vi "Refresh.vi"(0 "reference in":refnum<class "LcPictureBox.lvclass">, 5 "Error In":errorcluster) -> (14 "reference out":refnum<class "LcPictureBox.lvclass">, 19 "Error Out":errorcluster)   [LabVIEW 2020, in "LcPictureBox.lvclass"]
uses:
  LcPictureBox.lvclass
  System.Windows.Forms
  System.Drawing
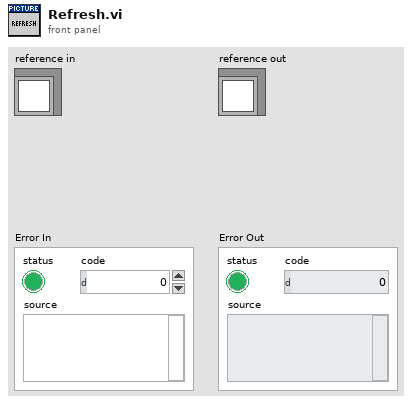
[diagram p1: front panel]
types:
  T1 = typedef "LcPictureBox.lvclass/ObjectAttributes.ctl" = cluster{"PictureBox":refnum<k24>, "ImageSize":cluster{"Width":i32, "Height":i32}, "PenMemory":map{cluster{"Alpha(100%)":dbl, "Color(Black)":u32, "Pen(Width=1, Solid)":T2}, refnum<k24>}, "GraphicsRef":refnum<k24>, "BrushMemory":map{cluster{"Alpha(100%)":dbl, "Color(Black)":u32}, refnum<k24>}, "Images":refnum<k24>[], "ImageIndex":i32, "BgColor(None)":u32, "LoadedImages":map{string, cluster{"ImageOut":refnum<k24>, "ImageSize":cluster{"Width":i32, "Height":i32}}}, "ColorsMemory":map{cluster{"Alpha(100%)":dbl, "Color(Black)":u32}, refnum<k24>}, "CacheSize":i32, "PictureBoxActiveXReference":refnum<vi>, "Scale":sgl, "Offset":cluster{"x":sgl, "y":sgl}, "zoom_center":cluster{"X":i32, "Y":i32}, "ImagesCreated":refnum<k24>[]}
  T2 = typedef "LcPictureBox.lvclass/Pen.ctl" = cluster{"Width":u16, "Style":enum32{"Solid", "Dash", "Dot", "DashDot", "DashDotDot"}}
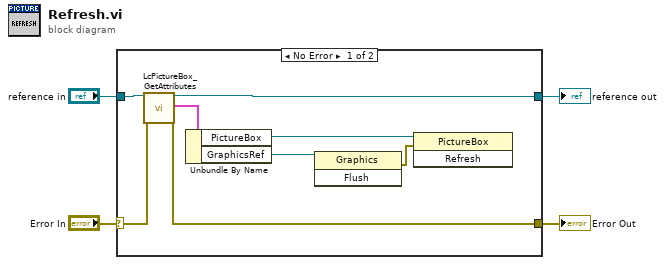
[diagram p0: block diagram]
diagram:
  n1 = case shown="No Error" "Error In" {
    selector: "Error In" -> [w12 w14]
    tunnel: [w10 w14] -> w3
    tunnel: [w8 w13] -> w1
    tunnel: "reference in" -> [w9 w13]
    frame No Error {
      n2 = call "LcPictureBox_GetAttributes.vi"("reference in"=w9, "error in (no error)"=w12) -> ("reference out"=w8:refnum<class "LcPictureBox.lvclass">, "Data"=w11:T1, "error out"=w10:errorcluster)  [unwired: 14 in, 1 out]
      n3 = Unbundle By Name(w11) -> ("PictureBox"=w7:refnum<k24>, "GraphicsRef"=w6:refnum<k24>)
      n4 = invoke class="Graphics" method="Flush"(reference=w6) -> (error out=w5:errorcluster)  [unwired: 2 in, 2 out]
      n5 = invoke class="PictureBox" method="Refresh"(reference=w7, error in=w5) -> ()  [unwired: 1 in, 3 out]
    }
    frame Error {
    }
  }
  "Error Out" <- w3
  "reference out" <- w1
